vi "W_b_init.vi"(2 "m":i32, 3 "n_l-1":i32, 4 "n_l":i32) -> (0 "b_l":T1, 1 "W_l":T1)   [LabVIEW 2016]
uses:
  <vilib>/Analysis/Matrix/Datatypes/RealMatrix.ctl
  <vilib>/Analysis/Matrix/Numeric/Conversions/Array To Matrix - RA2.vi
  <vilib>/Analysis/Matrix/NI_Matrix.lvlib
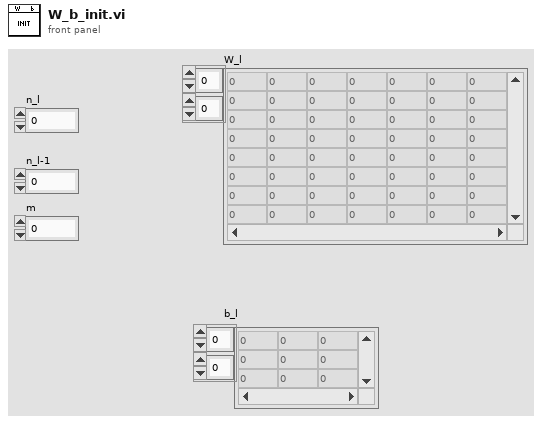
[diagram p1: front panel]
types:
  T1 = typedef "NI_Matrix.lvlib/RealMatrix.ctl" = dbl[][]
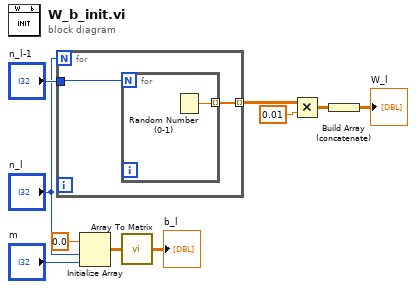
[diagram p0: block diagram]
diagram:
  n1 = for {
    N: "n_l" -> [_]
    tunnel: [w12] -> w2 mode=indexing
    tunnel: "n_l-1" -> [w11]
    n2 = for {
      N: w11 -> [_]
      tunnel: [w13] -> w12 mode=indexing
      n3 = Random Number (0-1)() -> (number: 0 to 1=w13:dbl)
    }
  }
  n4 = Initialize Array(0.0 ("element"), "n_l", "m") -> (w4:dbl[][])
  n5 = call-poly <vilib>:"Array To Matrix.vi"("Real 2D Array"=w4) -> ("Real Matrix"=→"b_l":T1)
  n6 = Multiply(x=w2, y=0.01) -> (x*y=w1:dbl[][])
  n7 = Build Array (concatenate)(w1) -> (→"W_l":T1)
